vi "Deconvolution.vi"(5 "DeconChannel":enum32{"No Selection", "Ch1", "Ch2", "Ch3"}(ring), 7 "iRF align":bool, 8 "error in (no error)":errorcluster, 11 "Waveform":dbl[](array[numeric])) -> (0 "error out":errorcluster, 2 "lifetime (ns)":dbl, 3 "Fitting":dbl[](array[numeric]))   [LabVIEW 2020]
uses:
  LaguerreDeconLib/DeconEngineClass/LaguerreDeconEngineClass.lvclass
  LaguerreDeconLib/DeconEngineClass/LaguerreDeconEngineClass.lvclass/LaguerreDeconEngineClass.ctl
panel:
  out "Waveform Graph":dbl[](graph)
  # "save the button here in case of future use"
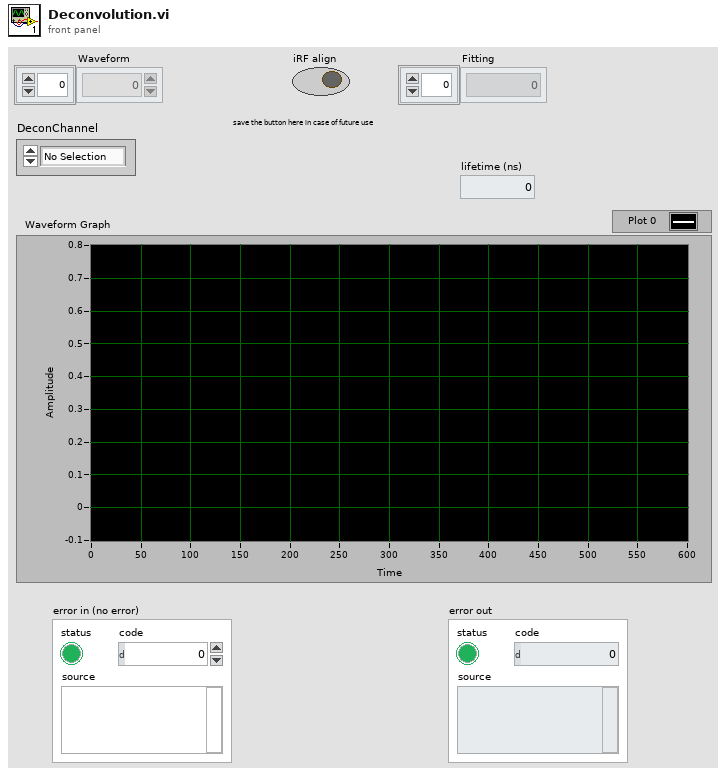
[diagram p1: front panel]
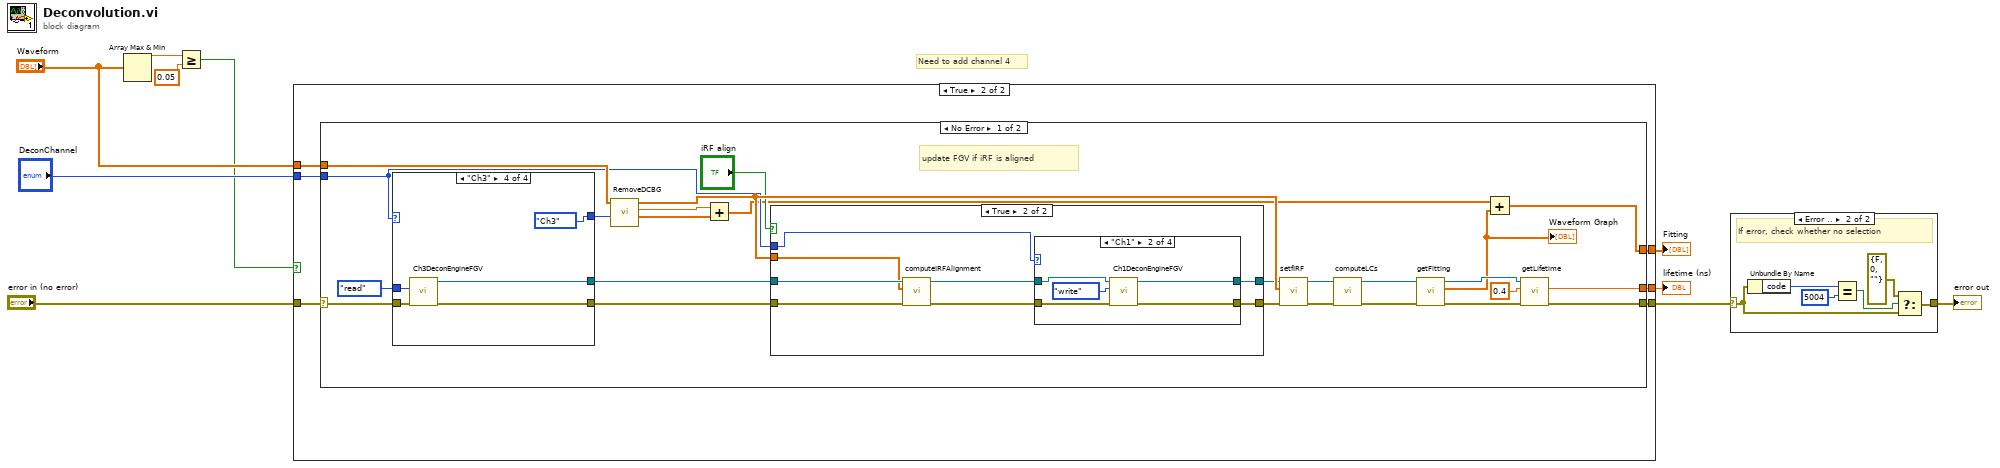
[diagram p0: block diagram]
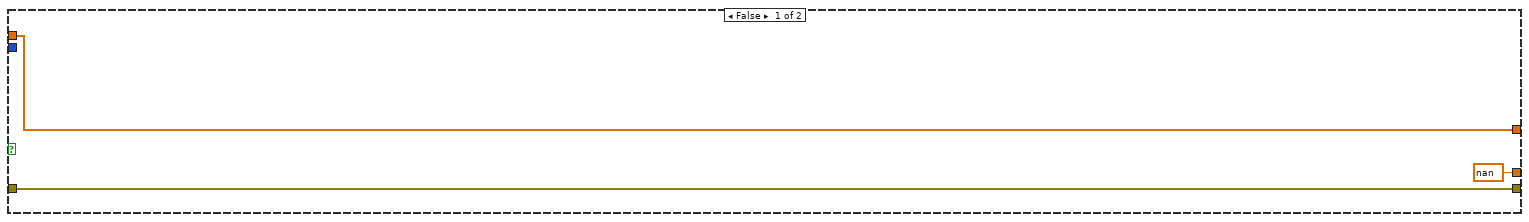
[diagram p2: hidden frame]
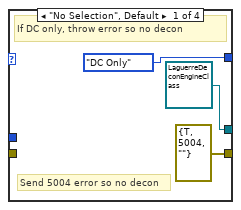
[diagram p3: hidden frame]
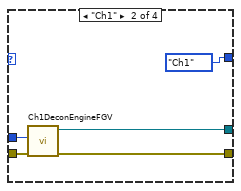
[diagram p4: hidden frame]
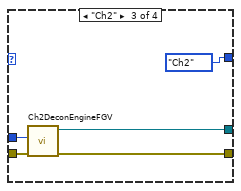
[diagram p5: hidden frame]
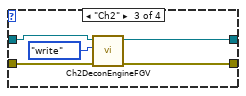
[diagram p8: hidden frame]
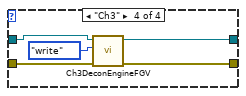
[diagram p9: hidden frame]
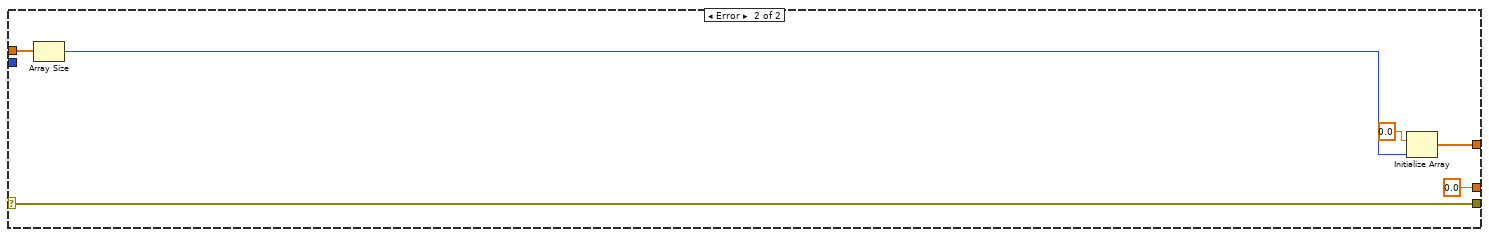
[diagram p10: hidden frame]
diagram:
  # "Need to add channel 4"
  n1 = Array Max & Min(array="Waveform") -> (max value=w3:dbl)  [unwired: 3 out]
  n2 = Greater Or Equal?(x=w3, y=0.05) -> (x >= y?=w1:bool)
  n3 = case shown="True" w1 {
    tunnel: [w13 w19] -> w10
    tunnel: [nan ("lifetime (ns)") w18] -> w9
    tunnel: "error in (no error)" -> [w11 w17]
    tunnel: "DeconChannel" -> [_ w16]
    tunnel: [w11 w15] -> w5
    tunnel: "Waveform" -> [w13 w14]
    frame False {
    }
    frame True {
      n4 = case shown="No Error" w17 {
        selector: w17 -> [w26 w95]
        tunnel: [w43 w95] -> w15
        tunnel: w14 -> [w29 w93]
        tunnel: [w28 w90] -> w19
        tunnel: [w27 0.0 ("lifetime (ns)")] -> w18
        tunnel: w16 -> [w25 _]
        frame No Error {
          # "update FGV if iRF is aligned"
          n5 = case shown="\"Ch3\"" w25 {
            tunnel: [errorcluster {"status"=TRUE, "code"=5004, "source"=""} ("Error Out") w52 w55 w60] -> w37
            tunnel: [refnum<class "LaguerreDeconEngineClass.lvclass"> refnum ("Ch3DeconEngine out") w51 w56 w59] -> w31
            tunnel: enum16{"write", "read"}."read" ("action") -> [_ w50 w54 w61]
            tunnel: w26 -> [_ w49 w57 w62]
            tunnel: [enum16{"DC Only", "Ch1", "Ch2", "Ch3"}."DC Only" ("Channel") enum16{"DC Only", "Ch1", "Ch2", "Ch3"}."Ch1" ("Channel") enum16{"DC Only", "Ch1", "Ch2", "Ch3"}."Ch2" ("Channel") enum16{"DC Only", "Ch1", "Ch2", "Ch3"}."Ch3" ("Channel")] -> w24
            frame "No Selection", Default {
              # "Send 5004 error so no decon"
              # "If DC only, throw error so no decon"
            }
            frame "Ch1" {
              n6 = call "Ch1DeconEngineFGV.vi"("Error In"=w49, "action(read)"=w50) -> ("Error Out"=w52:errorcluster, "Ch1DeconEngine out"=w51:refnum<class "LaguerreDeconEngineClass.lvclass">)  [unwired: 8 in]
            }
            frame "Ch2" {
              n7 = call "Ch2DeconEngineFGV.vi"("Error In"=w57, "action(read)"=w54) -> ("Error Out"=w55:errorcluster, "Ch2DeconEngine out"=w56:refnum<class "LaguerreDeconEngineClass.lvclass">)  [unwired: 8 in]
            }
            frame "Ch3" {
              n8 = call "Ch3DeconEngineFGV.vi"("Error In"=w62, "action(read)"=w61) -> ("Error Out"=w60:errorcluster, "Ch3DeconEngine out"=w59:refnum<class "LaguerreDeconEngineClass.lvclass">)  [unwired: 8 in]
            }
          }
          n9 = call "RemoveDCBG.vi"("Channel"=w24, "WF in"=w29) -> ("Scaled BG"=w21:dbl[], "DC"=w22:dbl, "WF out"=w38:dbl[])  [unwired: 7 in]
          n10 = Add(x=w22, y=w21) -> (x+y=w23:dbl[])
          n11 = case shown="True" "iRF align" {
            tunnel: w31 -> [w64 w72]
            tunnel: [w64 w66] -> w33
            tunnel: w38 -> [_ w71]
            tunnel: [w63 w67] -> w36
            tunnel: w37 -> [w63 w70]
            tunnel: w25 -> [_ w65]
            frame False {
            }
            frame True {
              n12 = call "computeIRFAlignment.vi"("error in (no error)"=w70, "fIRF temp"=w71, "LaguerreDeconEngineClass in"=w72) -> ("error out"=w68:errorcluster, "LaguerreDeconEngineClass out"=w69:refnum<class "LaguerreDeconEngineClass.lvclass">)  [unwired: 6 in, 1 out]
              n13 = case shown="\"Ch1\"" w65 {
                tunnel: w69 -> [w73 w78 w84 w89]
                tunnel: w68 -> [w74 w77 w82 w87]
                tunnel: [w74 w76 w81 w85] -> w67
                tunnel: [w73 w75 w83 w86] -> w66
                frame "No Selection", Default {
                }
                frame "Ch1" {
                  n14 = call "Ch1DeconEngineFGV.vi"("Error In"=w77, "action(read)"=enum16{"write", "read"}."write" ("action"), "Ch1DeconEngine in"=w78) -> ("Error Out"=w76:errorcluster, "Ch1DeconEngine out"=w75:refnum<class "LaguerreDeconEngineClass.lvclass">)  [unwired: 7 in]
                }
                frame "Ch2" {
                  n15 = call "Ch2DeconEngineFGV.vi"("Error In"=w82, "action(read)"=enum16{"write", "read"}."write" ("action"), "Ch2DeconEngine in"=w84) -> ("Error Out"=w81:errorcluster, "Ch2DeconEngine out"=w83:refnum<class "LaguerreDeconEngineClass.lvclass">)  [unwired: 7 in]
                }
                frame "Ch3" {
                  n16 = call "Ch3DeconEngineFGV.vi"("Error In"=w87, "action(read)"=enum16{"write", "read"}."write" ("action"), "Ch3DeconEngine in"=w89) -> ("Error Out"=w85:errorcluster, "Ch3DeconEngine out"=w86:refnum<class "LaguerreDeconEngineClass.lvclass">)  [unwired: 7 in]
                }
              }
            }
          }
          n17 = call "setfIRF.vi"("error in (no error)"=w36, "fIRF"=w38, "LaguerreDeconEngineClass in"=w33) -> ("error out"=w35:errorcluster, "LaguerreDeconEngineClass out"=w34:refnum<class "LaguerreDeconEngineClass.lvclass">)  [unwired: 7 in]
          n18 = call "computeLCs.vi"("error in (no error)"=w35, "LaguerreDeconClass in"=w34) -> ("error out"=w40:errorcluster, "LaguerreDeconClass out"=w39:refnum<class "LaguerreDeconEngineClass.lvclass">)  [unwired: 8 in]
          n19 = call "getFitting.vi"("error in (no error)"=w40, "LaguerreDeconEngineClass in"=w39) -> ("error out"=w42:errorcluster, "Fitting"=w20:dbl[], "LaguerreDeconEngineClass out"=w41:refnum<class "LaguerreDeconEngineClass.lvclass">)  [unwired: 7 in]
          "Waveform Graph" <- w20
          n20 = Add(x=w23, y=w20) -> (x+y=w28:dbl[])
          n21 = call "getLifetime.vi"("error in (no error)"=w42, "dt (ns)"=0.4, "LaguerreDeconEngineClass in"=w41) -> ("error out"=w43:errorcluster, "lifetime (ns)"=w27:dbl)  [unwired: 6 in, 1 out]
        }
        frame Error {
          n22 = Array Size(array=w93) -> (size(s)=w92:i32)
          n23 = Initialize Array(0.0 ("element"), w92) -> (w90:dbl[])
        }
      }
    }
  }
  "Fitting" <- w10
  "lifetime (ns)" <- w9
  n24 = case shown="Error .." w5 {
    selector: w5 -> [w96 w99]
    tunnel: [w96 w97] -> w6
    frame No Error {
      # "No error"
    }
    frame Error {
      # "If error, check whether no selection"
      n25 = Unbundle By Name(w99) -> ("code"=w102:i32)
      n26 = Equal?(x=w102, y=5004) -> (x = y?=w100:bool)
      n27 = Select(t=errorcluster {"status"=FALSE, "code"=0, "source"=""}, s=w100, f=w99) -> (s? t:f=w97:errorcluster)
    }
  }
  "error out" <- w6
